vi "Scanned Read - Mixed Module.vi"(6 "Mixed IO in":T1, 7 "Channel Type":T3, 8 "error in (no error)":errorcluster, 11 "IOV ref in":T2) -> (0 "error out":errorcluster, 3 "IOV ref out":T2, 4 "Mixed IO out":T1)   [LabVIEW 2019, in "SEECD Engine.lvlib"]
uses:
  SEECD Engine.lvlib
  Modules.lvlibp/RSI Module/Channel Type.ctl
  Type Defs/Open Module IOVs.ctl
  Type Defs/Mixed IO.ctl
  Modules.lvlibp/RSI Module/RSI Module.lvclass
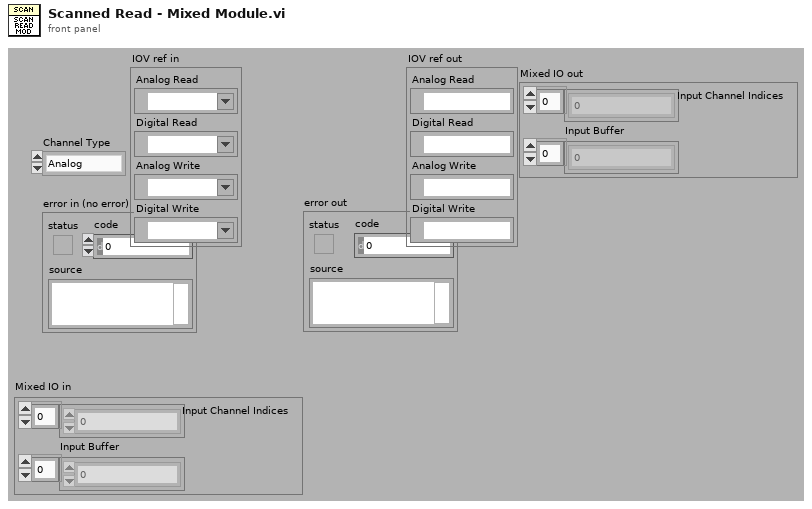
[diagram p1: front panel]
types:
  T1 = typedef "SEECD Engine.lvlib/Mixed IO.ctl" = cluster{"Input Channel Indices":i32[], "Input Buffer":dbl[]}
  T2 = typedef "SEECD Engine.lvlib/Open Module IOVs.ctl" = cluster{"Analog Read":refnum<k21>, "Digital Read":refnum<k21>, "Analog Write":refnum<k21>, "Digital Write":refnum<k21>}
  T3 = typedef "Modules.lvlibp/RSI Module.lvclass/Channel Type.ctl" = enum16{"Analog", "Digital"}
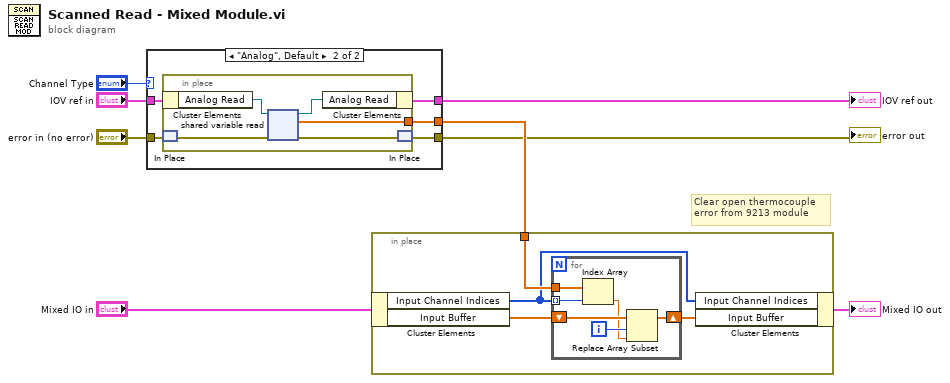
[diagram p0: block diagram]
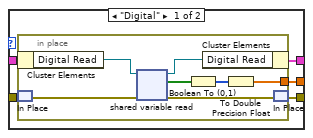
[diagram p2: hidden frame]
diagram:
  # "Clear open thermocouple\nerror from 9213 module"
  n1 = case shown="\"Analog\", Default" "Channel Type" {
    tunnel: "IOV ref in" -> [w13 w25]
    tunnel: "error in (no error)" -> [w10 w23]
    tunnel: [w9 w22] -> w1
    tunnel: [w12 w24] -> w4
    tunnel: [w11 w21] -> w5
    frame "Digital" {
      n2 = in-place {
        in-place-border: [w16] -> w11
        n3 = in-place-cluster #1(w13) -> ("Digital Read"=w20:refnum<k21>)
        n4 = in-place-match #2(w10) -> (w15:errorcluster)
        n5 = shared-variable-read(w20, w15) -> (w19:refnum<k21>, w14:errorcluster, w17:bool[])
        n6 = Boolean To (0,1)(Boolean=w17) -> (0, 1=w18:i16[])
        n7 = in-place-cluster #1("Digital Read"=w19) -> (w12:T2)
        n8 = To Double Precision Float(number=w18) -> (double precision float=w16:dbl[])
        n9 = in-place-match #2(w14) -> (w9:errorcluster)
      }
    }
    frame "Analog", Default {
      n10 = in-place {
        in-place-border: [w28] -> w21
        n11 = in-place-cluster #3(w25) -> ("Analog Read"=w30:refnum<k21>)
        n12 = in-place-match #4(w23) -> (w27:errorcluster)
        n13 = shared-variable-read(w30, w27) -> (w29:refnum<k21>, w26:errorcluster, w28:dbl[])
        n14 = in-place-cluster #3("Analog Read"=w29) -> (w24:T2)
        n15 = in-place-match #4(w26) -> (w22:errorcluster)
      }
    }
  }
  "error out" <- w1
  "IOV ref out" <- w4
  n16 = in-place {
    in-place-border: w5 -> [w34]
    n17 = in-place-cluster #5("Mixed IO in") -> ("Input Channel Indices"=w32:i32[], "Input Buffer"=w33:dbl[])
    n18 = for {
      tunnel: w32 -> [w39] mode=indexing
      tunnel: w34 -> [w40]
      shift-right: [w35] -> w31
      shift-left: w33 -> [w38]
      i -> [w37]
      n19 = Index Array(array=w40, index=w39) -> (element=w36:dbl)
      n20 = Replace Array Subset(array=w38, new element=w36, index=w37) -> (w35:dbl[])
    }
    n21 = in-place-cluster #5("Input Channel Indices"=w32, "Input Buffer"=w31) -> (→"Mixed IO out":T1)
  }
